vi "remove_HGFAgent.vi"(0 "MoAgSy_Engine.lvclass in":refnum<class "MoAgSy_Engine.lvclass">, 5 "error in (no error)":errorcluster) -> (14 "MoAgSy_Engine.lvclass out":refnum<class "MoAgSy_Engine.lvclass">, 15 "VarManagerEvent":refnum<class "HGF_Event.lvclass">, 16 "HGF_Event (Monitor Event)":refnum<class "HGF_Event.lvclass">, 17 "HGF_Agent":refnum<class "MoAgSy_AgentBase.lvclass">, 18 "Agent ID":string, 19 "error out":errorcluster)   [LabVIEW 2009, in "MoAgSy.lvlib" / "MoAgSy_Engine.lvclass"]
uses:
  MoAgSy_Engine.lvclass
  MoAgSy_AgentBase/MoAgSy_AgentBase.lvclass
  HGF_BaseClasses/HGF_Event/HGF_Event.lvclass
  MoAgSy_Engine.lvclass/MoAgSy_Engine.ctl
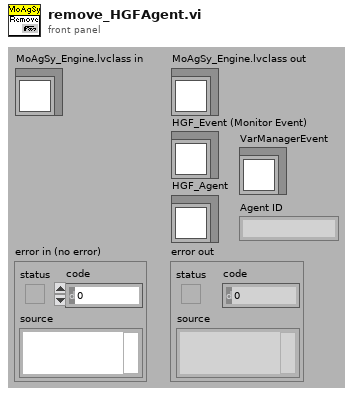
[diagram p1: front panel]
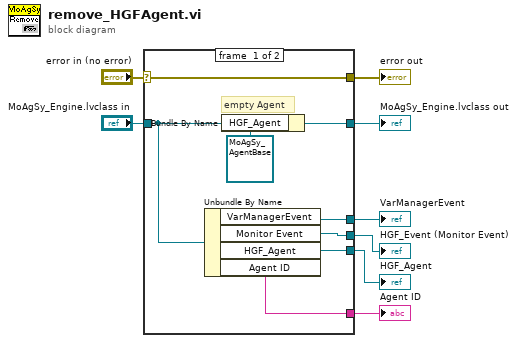
[diagram p0: block diagram]
diagram:
  n1 = case shown="No Error" "error in (no error)" {
    selector: "error in (no error)" -> [w16 w17]
    tunnel: [w16 w17] -> w7
    tunnel: [w13 w18] -> w5
    tunnel: "MoAgSy_Engine.lvclass in" -> [w15 w18]
    tunnel: [w14 _] -> w4
    tunnel: [w11 _] -> w3
    tunnel: [w10 _] -> w2
    tunnel: [w9 _] -> w1
    frame #0 {
      # "empty Agent"
      n2 = Unbundle By Name(w15) -> ("VarManagerEvent"=w9:refnum<class "HGF_Event.lvclass">, "Monitor Event"=w10:refnum<class "HGF_Event.lvclass">, "HGF_Agent"=w14:refnum<class "MoAgSy_AgentBase.lvclass">, "Agent ID"=w11:string)
      n3 = Bundle By Name(cluster=w15, "HGF_Agent"=refnum<class "MoAgSy_AgentBase.lvclass"> refnum) -> (w13:refnum<class "MoAgSy_Engine.lvclass">)
    }
    frame #1 {
    }
  }
  "error out" <- w7
  "MoAgSy_Engine.lvclass out" <- w5
  "HGF_Agent" <- w4
  "Agent ID" <- w3
  "HGF_Event (Monitor Event)" <- w2
  "VarManagerEvent" <- w1
